vi "FTW-Actor-Log-NewLog.vi"(0 "FTW Actor Instance":refnum<class "FTW-ActorInstance.lvclass">, 11 "error in":errorcluster) -> (4 "FTW Actor Instance out":refnum<class "FTW-ActorInstance.lvclass">, 8 "New Log File":path, 15 "error out":errorcluster)   [LabVIEW 2015, in "FTW-ActorInstance.lvclass"]
uses:
  FTW-ActorInstance.lvclass
  FTW-ActorInstance.lvclass/FTW-ActorInstance.ctl
  EventLogger/FTW-Logger.lvclass
panel:
  # "Inputs"
  # "Outputs"
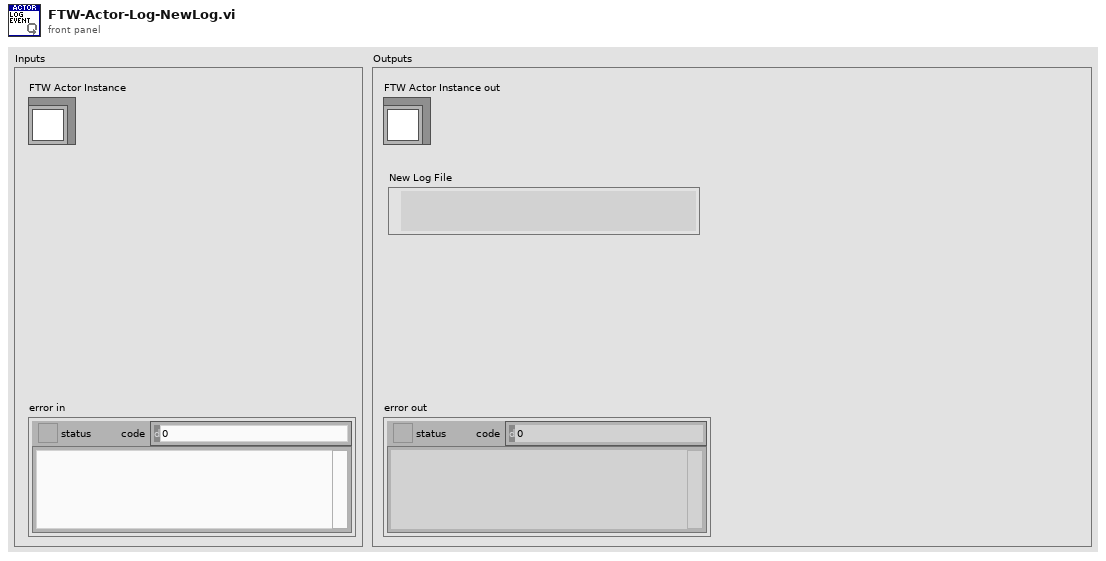
[diagram p1: front panel]
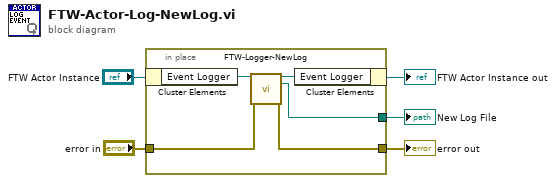
[diagram p0: block diagram]
diagram:
  n1 = in-place {
    in-place-border: "error in" -> [w10]
    in-place-border: [w7] -> w3
    in-place-border: [w6] -> w1
    n2 = in-place-cluster #1("FTW Actor Instance") -> ("Event Logger"=w9:refnum<class "FTW-Logger.lvclass">)
    n3 = call "FTW-Logger-NewLog.vi"("FTW Logger Connector"=w9, "error in"=w10) -> ("FTW Logger Connector out"=w8:refnum<class "FTW-Logger.lvclass">, "New Log File"=w7:path, "error out"=w6:errorcluster)  [unwired: 11 in]
    n4 = in-place-cluster #1("Event Logger"=w8) -> (→"FTW Actor Instance out":refnum<class "FTW-ActorInstance.lvclass">)
  }
  "error out" <- w1
  "New Log File" <- w3
